vi "gate sts.vi"(4 "Store\nTemperatures?":bool, 5 "?":bool, 6 "Store\nLock-in\nParameters?":bool, 7 "Stop":bool, 9 "End Gate (V)":dbl, 10 "Start Gate (V)":dbl, 11 "Basename":string) -> (3 "Current Gate Voltage (V)":dbl)   [LabVIEW 2021]
uses:
  <userlib>/Nanonis Prog Interface V5/Nanonis Prog Interface.lvlib
panel:
  in  "?":enum32{"Main", "Options", "Loop"}(tab)
  in  "Increment Gate (V)":dbl
  in  "Store\nMagnetic Field?":bool
  in  "Zigzag Raster?":bool
  in  "Insert Loop Index\ninto Basename?":bool
  in  "Loop Forever?":bool
  out "Loop Index":i32
  in  "Loop Index Offset":i32=1
  out "Ender":bool
  out "Stop Loop":bool
  # "Gate STS"
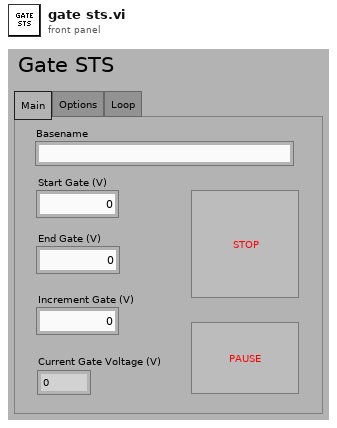
[diagram p1: front panel]
types:
  T1 = cluster{"Save all":enum16{"no change", "on", "off"}, "Number of Sweeps (0=no change)":i32}
  T2 = enum16{"Read State", "Hold", "Ramp to Set", "Ramp to Zero", "Read Switch Heater", "Switch Heater On", "Switch Heater Off", "Read Voltage", "Read Current", "Read Field", "Read Persistent Field", "Read Target Field", "Set Target Field", "Read Ramp Rate", "Set Ramp Rate"}
  T3 = enum16{"pot_temp", "sorb_temp", "needle_valve_temp", "still_temp", "mix_chamber_temp", "stm_rx_temp", "stm_cx_temp", "tank_pressure", "condense_pressure", "still_pressure", "turbo_back_pressure", "n2_trap_pressure"}
  T4 = enum16{"Set Amplitude", "Get Amplitude", "Set Frequency", "Get Frequency", "Set Harmonic", "Get Harmonic", "Set Phase", "Get Phase", "Auto Phase", "Add to Phase", "Autogain", "Set Time Constant", "Get Time Constant", "Set Sensitivity", "Get Sensitivity", "Set Input A", "Set Input A-B", "Get Input Setting", "Set Offset", "Get Offset"}[]
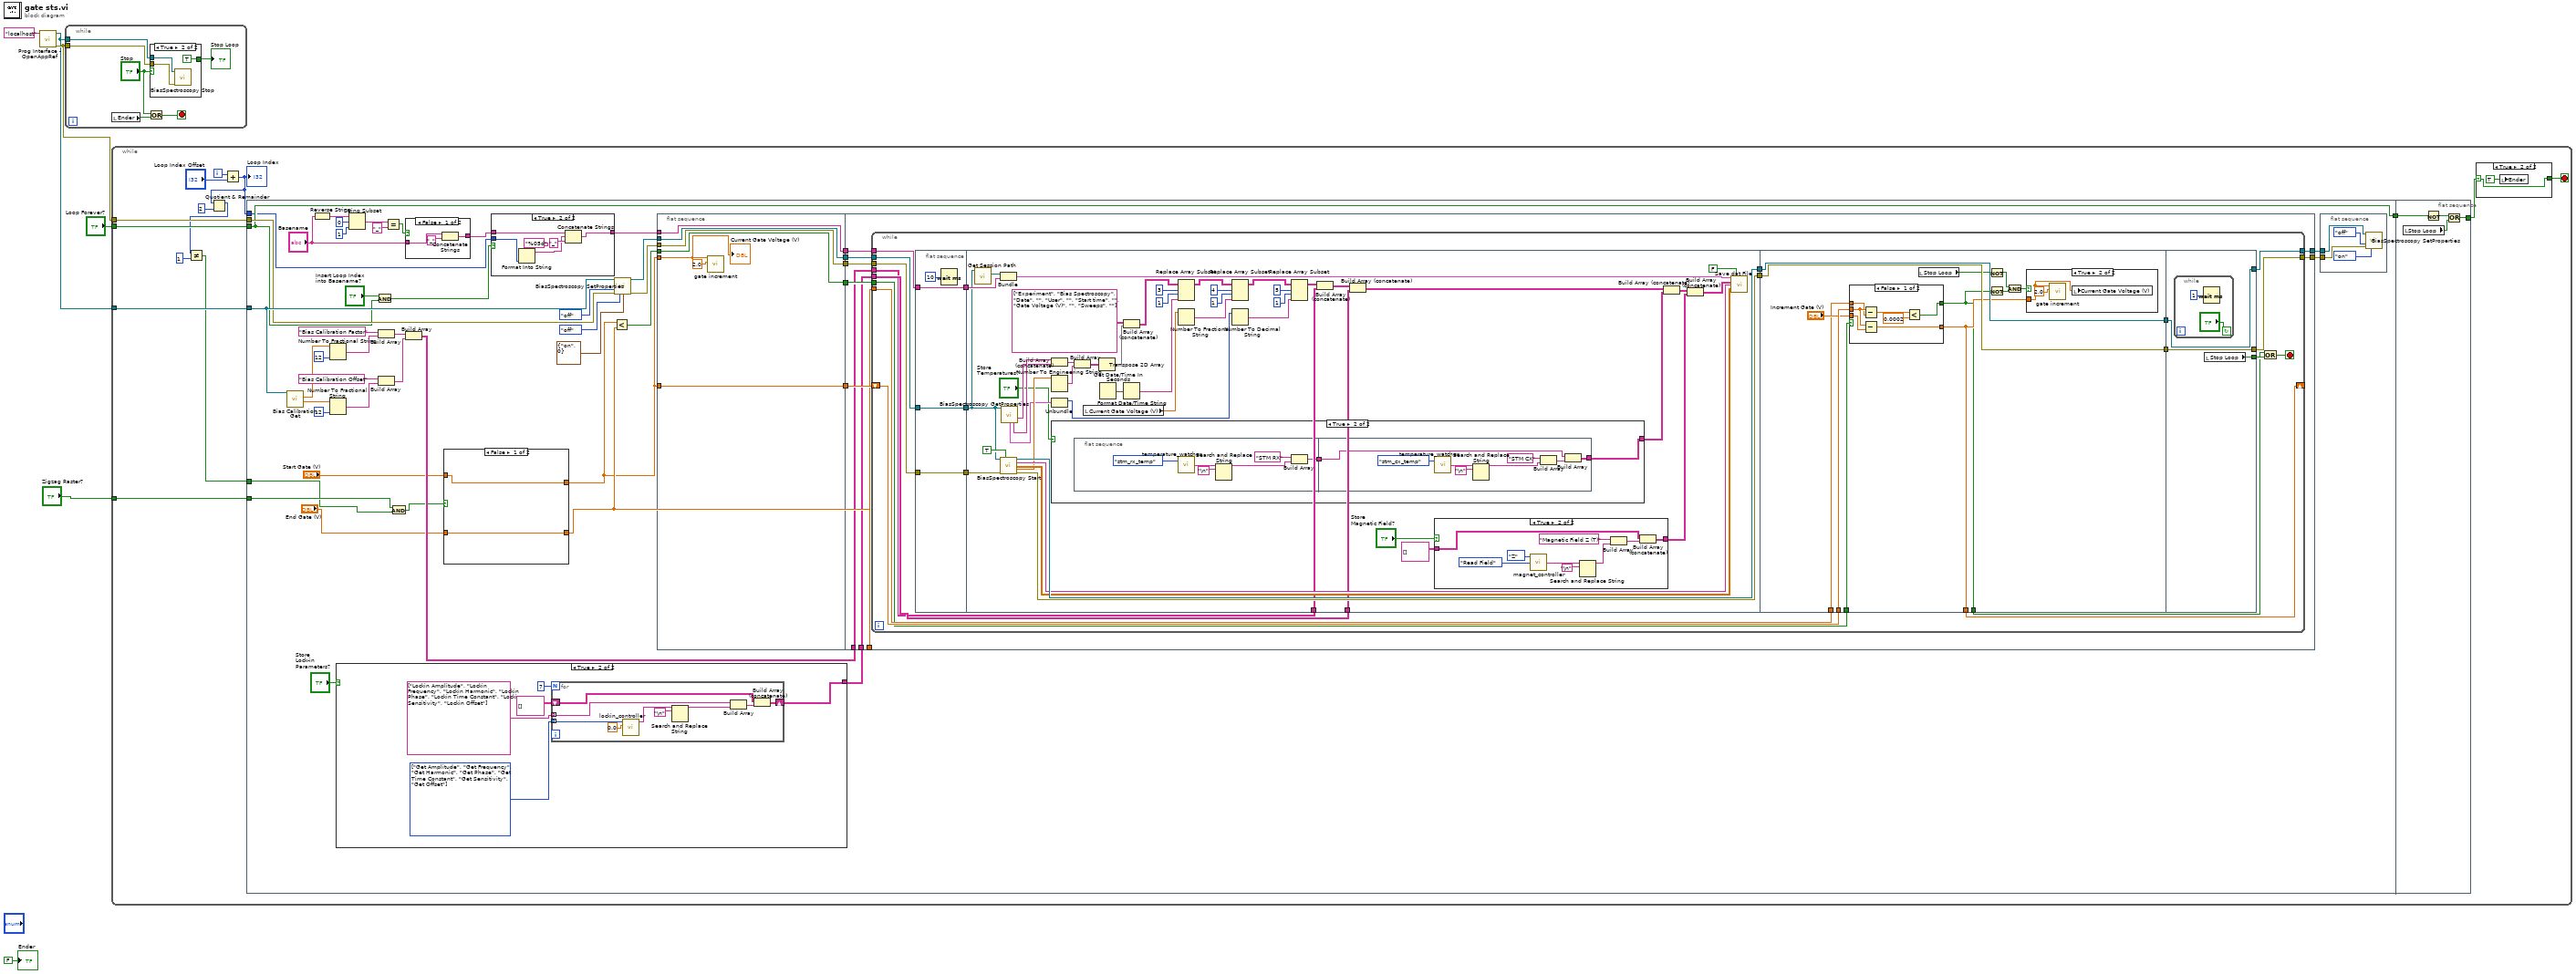
[diagram p0: block diagram]
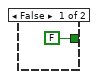
[diagram p2: hidden frame]
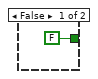
[diagram p3: hidden frame]
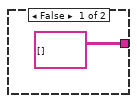
[diagram p7: hidden frame]
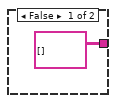
[diagram p9: hidden frame]
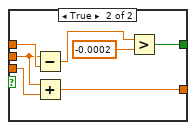
[diagram p10: hidden frame]
diagram:
  n1 = call <userlib>:"Prog Interface - OpenAppRef.vi"("Machine name (local machine IP)"="localhost" ("machine name (localhost)")) -> ("Error out"=w3:errorcluster, "Application reference"=w2:refnum<vi>)  [unwired: 5 in]
  n2 = while {
    tunnel: w2 -> [w12]
    tunnel: w3 -> [w11]
    stop <- w8 stop-if-true
    n3 = local read "Ender"() -> (w7:bool)
    n4 = Or(x="Stop", y=w7) -> (x .or. y?=w8:bool)
    n5 = case shown="True" "Stop" {
      tunnel: w12 -> [_ w16]
      tunnel: w11 -> [_ w15]
      tunnel: [FALSE TRUE] -> w10
      frame False {
      }
      frame True {
        n6 = call <userlib>:"BiasSpectroscopy Stop.vi"("Application ref in"=w16, "Error in (no error)"=w15) -> ()  [unwired: 12 in, 2 out]
      }
    }
    "Stop Loop" <- w10
  }
  n7 = while {
    tunnel: "Loop Forever?" -> [w30]
    tunnel: w2 -> [w28]
    tunnel: w3 -> [w27]
    tunnel: "Zigzag Raster?" -> [w23]
    i -> [w24]
    stop <- w25 stop-if-true
    n8 = Add(x=w24, y="Loop Index Offset") -> (x+y=w21:i32)
    "Loop Index" <- w21
    n9 = Quotient & Remainder(x=w21, y=2) -> (x-y*floor(x/y)=w19:i32)  [unwired: 1 out]
    n10 = Not Equal?(x=w19, y=1) -> (x != y?=w17:bool)
    n11 = flat-sequence {
      tunnel: w30 -> [w51]
      tunnel: [w51] -> w29
      tunnel: w28 -> [w55]
      tunnel: w27 -> [w54]
      tunnel: w21 -> [w49]
      tunnel: w23 -> [w36]
      tunnel: w17 -> [w35]
      tunnel: w29 -> [w268]
      tunnel: [w265] -> w26
      frame #0 {
        n12 = call <userlib>:"Bias Calibration Get.vi"("Application ref in"=w55) -> ("Offset (V)"=w65:sgl, "Calibration (V/V)"=w66:sgl)  [unwired: 7 in, 2 out]
        n13 = Reverse String(1:"Basename") -> (0:w46:string)
        n14 = Number To Fractional String(number=w66, precision (6)=i16 12) -> (F-format string=w62:string)  [unwired: 2 in]
        n15 = Number To Fractional String(number=w65, precision (6)=i16 12) -> (F-format string=w59:string)  [unwired: 2 in]
        n16 = case shown="True" "Store\nLock-in\nParameters?" {
          tunnel: [string[][] [] w98] -> w67
          frame False {
          }
          frame True {
            w101 = T4 [enum."Get Amplitude", enum."Get Frequency", enum."Get Harmonic", enum."Get Phase", enum."Get Time Constant", enum."Get Sensitivity", enum."Get Offset"] items=["Set Amplitude", "Get Amplitude", "Set Frequency", "Get Frequency", "Set Harmonic", "Get Harmonic", "Set Phase", "Get Phase", "Auto Phase", "Add to Phase", "Autogain", "Set Time Constant", "Get Time Constant", "Set Sensitivity", "Get Sensitivity", "Set Input A", "Set Input A-B", "Get Input Setting", "Set Offset", "Get Offset"]
            n17 = for {
              N: 7 -> [_]
              tunnel: w101 -> [w109] mode=indexing
              tunnel: string[] ["Lockin Amplitude", "Lockin Frequency", "Lockin Harmonic", "Lockin Phase", "Lockin Time Constant", "Lockin Sensitivity", "Lockin Offset"] -> [w108] mode=indexing
              shift-right: [w106] -> w98
              shift-left: string[][] [] -> [w107]
              n18 = call "lockin_controller.vi"("Numerical Argument"=0.0, "Command"=w109) -> ("Response"=w104:string)  [unwired: 9 in]
              n19 = Search and Replace String(input string=w104, search string="\n") -> (result string=w105:string)  [unwired: 6 in, 3 out]
              n20 = Build Array(w108, w105) -> (w110:string[])
              n21 = Build Array (concatenate)(w107, w110) -> (w106:string[][])
            }
          }
        }
        n22 = String Subset(string=w46, offset (0)=0, length (rest)=1 ("length (rest)")) -> (substring=w45:string)
        n23 = And(x="Insert Loop Index\ninto Basename?", y=w51) -> (x .and. y?=w50:bool)
        n24 = Build Array("Bias Calibration Factor" ("element"), w62) -> (w57:string[])
        n25 = Build Array("Bias Calibration Offset" ("element"), w59) -> (w58:string[])
        n26 = Equal?(x=w45, y="_") -> (x = y?=w43:bool)
        n27 = And(x=w36, y=w35) -> (x .and. y?=w34:bool)
        n28 = case shown="False" w43 {
          tunnel: "Basename" -> [w87 w89]
          tunnel: [w86 w89] -> w41
          frame False {
            n29 = Concatenate Strings(w87, "_" ("string")) -> (w86:string)
          }
          frame True {
          }
        }
        n30 = Build Array(w57, w58) -> (w56:string[][])
        n31 = case shown="False" w34 {
          tunnel: "End Gate (V)" -> [w83 w85]
          tunnel: [w83 w84] -> w39
          tunnel: [w82 w85] -> w38
          tunnel: "Start Gate (V)" -> [w82 w84]
          frame False {
          }
          frame True {
          }
        }
        n32 = case shown="True" w50 {
          tunnel: [w90 w96] -> w53
          tunnel: w41 -> [w90 w95]
          tunnel: w49 -> [_ w93]
          frame False {
          }
          frame True {
            n33 = Format Into String(format string="%05d", w93) -> (resulting string=w91:string)  [unwired: 2 in, 1 out]
            n34 = Concatenate Strings(w95, w91, "_" ("string")) -> (w96:string)
          }
        }
        n35 = Less?(x=w38, y=w39) -> (x < y?=w70:bool)
        n36 = call <userlib>:"BiasSpectroscopy SetProperties.vi"("Application ref in"=w55, "Autosave (no change)"=enum16{"no change", "on", "off"}."off", "Error in (no error)"=w54, "Save dialog"=enum16{"no change", "on", "off"}."off", "Multiple sweeps config"=T1 {"Save all"=enum."on", "Number of Sweeps (0=no change)"=0}) -> ("Application ref out"=w75:refnum<vi>, "Error out"=w76:errorcluster)  [unwired: 9 in]
        n37 = flat-sequence {
          tunnel: w38 -> [w118]
          tunnel: w70 -> [w119]
          tunnel: w75 -> [w120]
          tunnel: w76 -> [w121]
          tunnel: w53 -> [w122]
          tunnel: [w122] -> w81
          tunnel: [w121] -> w80
          tunnel: [w120] -> w79
          tunnel: [w119] -> w78
          tunnel: [w118] -> w77
          tunnel: w38 -> [w116]
          tunnel: [w129] -> w73
          tunnel: [w128] -> w72
          tunnel: w81 -> [w132]
          tunnel: w80 -> [w131]
          tunnel: w79 -> [w130]
          tunnel: w78 -> [w127]
          tunnel: w77 -> [w126]
          tunnel: w39 -> [w125]
          tunnel: w67 -> [w124]
          tunnel: w56 -> [w123]
          frame #0 {
            n38 = call "gate increment.vi"("Increment"=2.0, "Gate Voltage"=w116) -> ()  [unwired: 10 in]
            "Current Gate Voltage (V)" <- w116
          }
          frame #1 {
            n39 = while {
              tunnel: w132 -> [w153]
              tunnel: w131 -> [w152]
              tunnel: w130 -> [w151]
              tunnel: [w150] -> w129
              tunnel: [w149] -> w128
              tunnel: w127 -> [w135]
              shift-right: [w139] -> _
              shift-left: w126 -> [w137]
              tunnel: w125 -> [w136]
              tunnel: w124 -> [w134]
              tunnel: w123 -> [w133]
              stop <- w140 stop-if-true
              n40 = flat-sequence {
                tunnel: w151 -> [w155]
                tunnel: w152 -> [w156]
                tunnel: w153 -> [w157]
                tunnel: [w157] -> w144
                tunnel: [w156] -> w143
                tunnel: [w155] -> w142
                tunnel: [w202] -> w146
                tunnel: [w203] -> w145
                tunnel: w144 -> [w195]
                tunnel: w143 -> [w204]
                tunnel: w142 -> [w194]
                tunnel: w134 -> [w169]
                tunnel: w133 -> [w167]
                tunnel: [w243] -> w148
                tunnel: [w242] -> w147
                tunnel: w146 -> [w243]
                tunnel: w145 -> [w242]
                tunnel: [w238] -> w139
                tunnel: [w236] -> w138
                tunnel: w137 -> [w235]
                tunnel: w136 -> [w233]
                tunnel: w135 -> [w232]
                tunnel: [w261] -> w150
                tunnel: [w262] -> w149
                tunnel: w148 -> [w262]
                tunnel: w147 -> [w261]
                tunnel: [w260] -> w141
                frame #0 {
                  n41 = Wait (ms)(milliseconds to wait=u32 10) -> ()  [unwired: 1 out]
                }
                frame #1 {
                  n42 = call <userlib>:"Get Session Path.vi"("Application ref in"=w194) -> ("Session path"=w200:path)  [unwired: 8 in, 2 out]
                  n43 = Bundle("Session path"=w200, "Basename"=w195) -> (w199:cluster{"Session path":path, "Basename":string})  [unwired: 1 in]
                  n44 = call <userlib>:"BiasSpectroscopy Start.vi"("Application ref in"=w194, "Get data (F)"=TRUE, "Error in (no error)"=w204) -> ("Application ref out"=w203:refnum<vi>, "Channels"=w197:string[], "Data"=w198:sgl[][], "Parameters"=w193:sgl[], "Error out"=w202:errorcluster)  [unwired: 8 in]
                  n45 = call <userlib>:"BiasSpectroscopy GetProperties.vi"("Application ref in"=w194) -> ("Parameters"=w186:string[], "Multiple sweeps configuration"=w175:cluster{"Number of Sweeps":i32, "Save all":bool}, "Fixed parameters"=w187:string[])  [unwired: 7 in, 5 out]
                  n46 = Build Array (concatenate)(w187, w186) -> (w191:string[])
                  n47 = Number To Engineering String(4:w193) -> (0:w192:string[])  [unwired: 3 in]
                  n48 = Unbundle(w175) -> ("Number of Sweeps"=w174:i32)  [unwired: 1 out]
                  n49 = case shown="True" "Store\nTemperatures?" {
                    tunnel: [string[][] [] w216] -> w163
                    frame False {
                    }
                    frame True {
                      n50 = flat-sequence {
                        tunnel: [w221] -> w217
                        tunnel: w217 -> [w228]
                        tunnel: [w227] -> w216
                        frame #0 {
                          n51 = call "temperature_watcher.vi"("Command"=T3."stm_rx_temp") -> ("Response"=w219:string)  [unwired: 1 in]
                          n52 = Search and Replace String(input string=w219, search string="\n") -> (result string=w218:string)  [unwired: 6 in, 3 out]
                          n53 = Build Array("STM RX" ("element"), w218) -> (w221:string[])
                        }
                        frame #1 {
                          n54 = call "temperature_watcher.vi"("Command"=T3."stm_cx_temp") -> ("Response"=w225:string)  [unwired: 1 in]
                          n55 = Search and Replace String(input string=w225, search string="\n") -> (result string=w224:string)  [unwired: 6 in, 3 out]
                          n56 = Build Array("STM CX" ("element"), w224) -> (w229:string[])
                          n57 = Build Array(w228, w229) -> (w227:string[][])
                        }
                      }
                    }
                  }
                  n58 = Build Array(w191, w192) -> (w190:string[][])
                  n59 = local read "Current Gate Voltage (V)"() -> (w177:dbl)
                  n60 = Transpose 2D Array(2D array=w190) -> (transposed array=w188:string[][])
                  n61 = Get Date/Time In Seconds() -> (seconds since 1Jan1904=w185:timestamp)
                  n62 = Build Array (concatenate)(string[][] [["Experiment", "Bias Spectroscopy"], ["Date", ""], ["User", ""], ["Start time", ""], ["Gate Voltage (V)", ""], ["Sweeps", ""]] ("Attributes"), w188) -> (w184:string[][])
                  n63 = Format Date/Time String(seconds (now)=w185) -> (date/time string=w183:string)  [unwired: 2 in]
                  n64 = Replace Array Subset(array=w184, new element=w183, index (row)=3, index (col)=1 ("disabled index (col)")) -> (w180:string[][])
                  n65 = Number To Fractional String(number=w177) -> (F-format string=w176:string)  [unwired: 3 in]
                  n66 = Replace Array Subset(array=w180, new element=w176, index (row)=4, index (col)=1 ("disabled index (col)")) -> (w173:string[][])
                  n67 = Number To Decimal String(number=w174) -> (decimal integer string=w170:string)  [unwired: 1 in]
                  n68 = Replace Array Subset(array=w173, new element=w170, index (row)=5, index (col)=1 ("disabled index (col)")) -> (w168:string[][])
                  n69 = Build Array (concatenate)(w168, w167) -> (w166:string[][])
                  n70 = Build Array (concatenate)(w166, w169) -> (w164:string[][])
                  n71 = case shown="True" "Store\nMagnetic Field?" {
                    tunnel: [w205 w209] -> w159
                    tunnel: string[][] [] ("array") -> [w205 w210]
                    frame False {
                    }
                    frame True {
                      n72 = call "magnet_controller.vi"("Command"=T2."Read Field", "Direction"=enum16{"X", "Y", "Z"}."Z") -> ("Response"=w207:string)  [unwired: 1 in]
                      n73 = Search and Replace String(input string=w207, search string="\n") -> (result string=w206:string)  [unwired: 6 in, 3 out]
                      n74 = Build Array("Magnetic Field Z (T)" ("element"), w206) -> (w211:string[])
                      n75 = Build Array (concatenate)(w210, w211) -> (w209:string[][])
                    }
                  }
                  n76 = Build Array (concatenate)(w164, w163) -> (w160:string[][])
                  n77 = Build Array (concatenate)(w160, w159) -> (w161:string[][])
                  n78 = call <userlib>:"Save dat File.vi"("Filename control"=w199, "Show save dialog (T)"=FALSE, "Attributes"=w161, "Channels names"=w197, "Data"=w198) -> ()  [unwired: 7 in, 4 out]
                }
                frame #2 {
                  n79 = case shown="False" w232 {
                    tunnel: w235 -> [w248 w254]
                    tunnel: "Increment Gate (V)" -> [w249 w257]
                    tunnel: [w250 w256] -> w238
                    tunnel: w233 -> [w247 w255]
                    tunnel: [w245 w253] -> w236
                    frame False {
                      n80 = Subtract(x=w248, y=w247) -> (x-y=w246:dbl)
                      n81 = Subtract(x=w248, y=w249) -> (x-y=w250:dbl)
                      n82 = Less?(x=w246, y=0.0002) -> (x < y?=w245:bool)
                    }
                    frame True {
                      n83 = Subtract(x=w254, y=w255) -> (x-y=w252:dbl)
                      n84 = Add(x=w254, y=w257) -> (x+y=w256:dbl)
                      n85 = Greater?(x=w252, y=-0.0002) -> (0:w253:bool)
                    }
                  }
                  n86 = local read "Stop Loop"() -> (w241:bool)
                  n87 = Not(x=w241) -> (.not. x?=w239:bool)
                  n88 = Not(x=w236) -> (.not. x?=w237:bool)
                  n89 = And(x=w239, y=w237) -> (x .and. y?=w240:bool)
                  n90 = case shown="True" w240 {
                    tunnel: w238 -> [_ w259]
                    frame False {
                    }
                    frame True {
                      n91 = call "gate increment.vi"("Increment"=2.0, "Gate Voltage"=w259) -> ()  [unwired: 10 in]
                      n92 = local write "Current Gate Voltage (V)"(w259) -> ()
                    }
                  }
                }
                frame #3 {
                  n93 = while {
                    stop <- "?" continue-if-true
                    n94 = Wait (ms)(milliseconds to wait=u32 1) -> ()  [unwired: 1 out]
                  }
                  n95 = local read "Stop Loop"() -> (w260:bool)
                }
              }
              n96 = Or(x=w138, y=w141) -> (x .or. y?=w140:bool)
            }
          }
        }
        n97 = flat-sequence {
          tunnel: w73 -> [w115]
          tunnel: w72 -> [w114]
          frame #0 {
            n98 = call <userlib>:"BiasSpectroscopy SetProperties.vi"("Application ref in"=w115, "Autosave (no change)"=enum16{"no change", "on", "off"}."off", "Error in (no error)"=w114, "Save dialog"=enum16{"no change", "on", "off"}."on") -> ()  [unwired: 10 in, 2 out]
          }
        }
      }
      frame #1 {
        n99 = local read "Stop Loop"() -> (w267:bool)
        n100 = Not(x=w268) -> (.not. x?=w266:bool)
        n101 = Or(x=w266, y=w267) -> (x .or. y?=w265:bool)
      }
    }
    n102 = case shown="True" w26 {
      selector: w26 -> [_ w33]
      tunnel: [FALSE w33] -> w25
      frame False {
      }
      frame True {
        n103 = local write "Ender"(TRUE ("Ender")) -> ()
      }
    }
  }
  "Ender" <- FALSE ("Ender")
